vi "Format Boolean Info for File.vi"(0 "File Name":path, 1 "Label Name":string, 2 "Time (msec)":u32, 3 "error in (no error)":errorcluster) -> (10 "error out":errorcluster)   [LabVIEW 2009]
doc: "This VI is a sub VI used in the drop ins exercise. \n\nAAL 9/09"
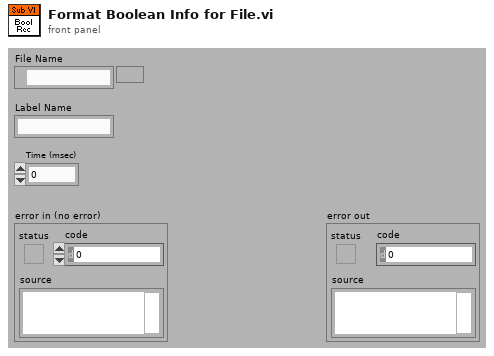
[diagram p1: front panel]
types:
  T1 = enum16{"open", "replace", "create", "open or create", "replace or create", "replace or create with confirmation"}
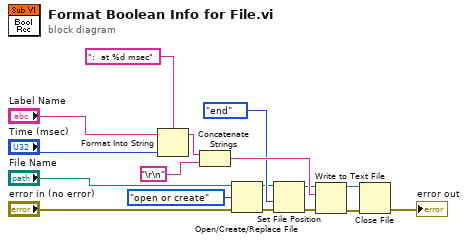
[diagram p0: block diagram]
diagram:
  n1 = Format Into String(format string=":  at %d msec", initial string="Label Name", "Time (msec)") -> (resulting string=w3:string)  [unwired: 1 in, 1 out]
  n2 = Concatenate Strings(w3, "\r\n") -> (w16:string)
  n3 = Open/Create/Replace File(file path (use dialog)="File Name", error in="error in (no error)", operation (0:open)=T1."open or create") -> (refnum out=w10:refnum<file>, error out=w9:errorcluster)  [unwired: 4 out]
  n4 = Set File Position(refnum=w10, from (0:start)=enum16{"start", "end", "current"}."end", error in=w9) -> (refnum out=w12:refnum<file>, error out=w11:errorcluster)  [unwired: 1 out]
  n5 = Write to Text File(file (use dialog)=w12, text=w16, error in=w11) -> (refnum out=w7:refnum<file>, error out=w6:errorcluster)  [unwired: 2 out]
  n6 = Close File(refnum=w7, error in=w6) -> (error out=→"error out":errorcluster)  [unwired: 1 out]
